vi "Data_Reader.vi"() -> ()   [LabVIEW 2017]
panel:
  out "Signal":dynamicdata(graph) caption="Sine"
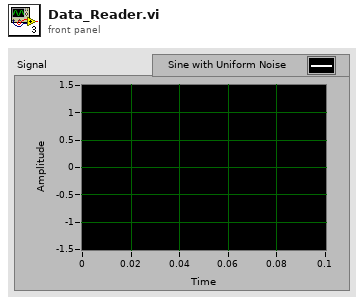
[diagram p1: front panel]
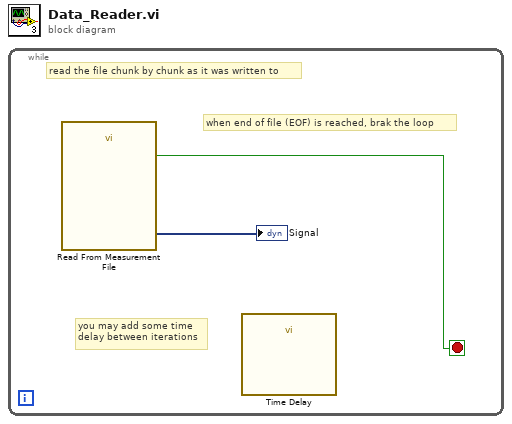
[diagram p0: block diagram]
diagram:
  n1 = while {
    stop <- w1 stop-if-true
    # "you may add some time\ndelay between iterations"
    # "when end of file (EOF) is reached, brak the loop"
    # "read the file chunk by chunk as it was written to"
    n2 = call "Read From Measurement File"() -> ("Signals"=→"Signal":dynamicdata, "EOF?"=w1:bool)  [unwired: 6 in, 4 out]
    n3 = call "Time Delay"() -> ()  [unwired: 11 in, 1 out]
  }
